vi "testCameraStack.vi"() -> ()   [LabVIEW 2015]
uses:
  <vilib>/userdefined/High Color/IMAQdx.ctl
  <vilib>/vision/driver/NI_Vision_Acquisition_Software.lvlib
  <resource>/objmgr/imaqdx.rc
panel:
  out "Classes (Color Classification 1) 2":string[](array[string])
  out "Classes (Color Classification 1)":string[](array[string])
  out "Image":T1(plugin-control)
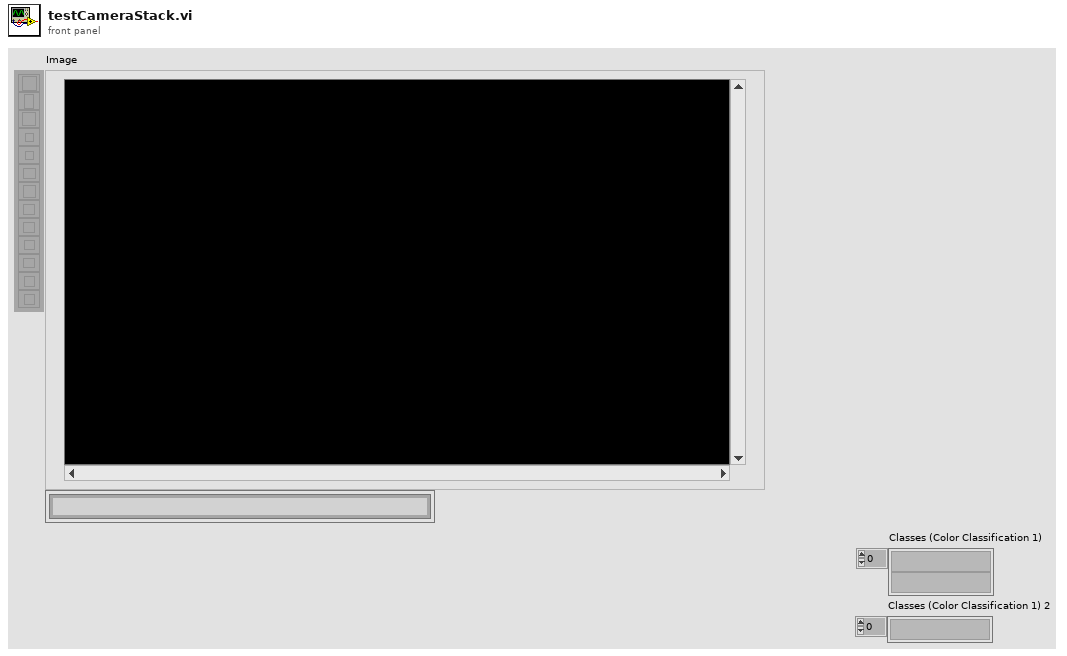
[diagram p1: front panel]
types:
  T1 = typedef "IMAQ Image.ctl" = refnum<image>
  T2 = typedef "IMAQdx.ctl" = refnum<k21>
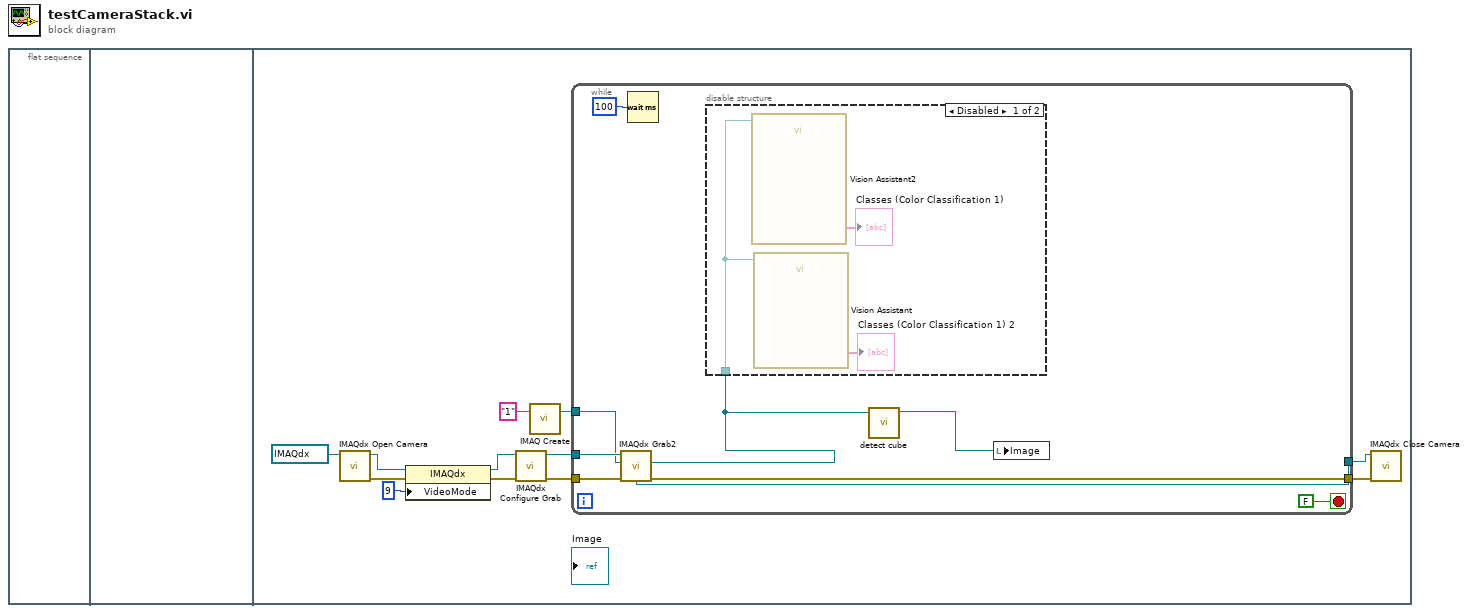
[diagram p0: block diagram]
diagram:
  n1 = flat-sequence {
    frame #0 {
    }
    frame #1 {
    }
    frame #2 {
      n2 = call <vilib>:"IMAQdx Open Camera.vi"("Session In"=T2 "cam2") -> ("error out"=w4:errorcluster, "Session Out"=w5:T2)  [unwired: 9 in]
      n3 = property class="IMAQdx"(reference=w5, error in=w4, "VideoMode"=u32 9) -> (reference out=w2:T2, error out=w3:errorcluster)
      n4 = call <vilib>:"IMAQdx Configure Grab.vi"("error in"=w3, "Session In"=w2) -> ("error out"=w11:errorcluster, "Session Out"=w10:T2)  [unwired: 8 in]
      n5 = call "IMAQ Create"("Image Name"="1") -> ("New Image"=w8:T1)  [unwired: 4 in, 1 out]
      n6 = while {
        tunnel: w11 -> [w21]
        tunnel: w10 -> [w20]
        tunnel: [w19] -> w9
        tunnel: w8 -> [w18]
        tunnel: [w17] -> w6
        stop <- FALSE stop-if-true
        n7 = call <vilib>:"IMAQdx Grab2.vi"("error in"=w21, "Image In"=w18, "Session In"=w20) -> ("error out"=w17:errorcluster, "Image Out"=w14:T1, "Session Out"=w19:T2)  [unwired: 5 in, 1 out]
        n8 = Wait (ms)(milliseconds to wait=u32 100) -> ()  [unwired: 1 out]
        n9 = disable-structure shown="Disabled" {
          disable-tunnel: w14 -> [w24 _]
          frame Disabled {
            n10 = call "Vision Assistant2"("Image In"=w24) -> ("Classes (Color Classification 1)"=→"Classes (Color Classification 1)":string[])  [unwired: 24 in, 2 out]
            n11 = call "Vision Assistant"("Image In"=w24) -> ("Classes (Color Classification 1)"=→"Classes (Color Classification 1) 2":string[])  [unwired: 24 in, 2 out]
          }
          frame Enabled {
          }
        }
        n12 = call "detect cube.vi"("Image 3"=w14) -> ("Image 4"=w13:T1)  [unwired: 2 in, 4 out]
        n13 = local write "Image"(w13) -> ()
      }
      n14 = call <vilib>:"IMAQdx Close Camera.vi"("error in"=w6, "Session In"=w9) -> ()  [unwired: 9 in, 1 out]
    }
  }
